vi "Shell.vi"(1 "b":dbl=2.0, 2 "a":dbl=4.0) -> (0 "result":dbl=4.0)   [LabVIEW 2019, in "lv-providershell-example1.lvlib"]
uses:
  lv-providershell-example1.lvlib
  src/VIProviderShellHelper.lvclass
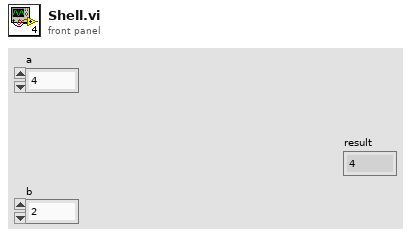
[diagram p1: front panel]
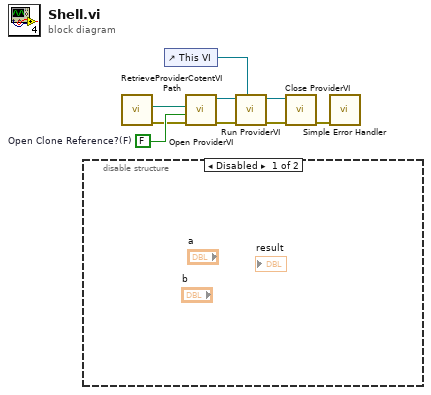
[diagram p0: block diagram]
diagram:
  w5 = FALSE  # Open Clone Reference?(F)
  n1 = disable-structure shown="Disabled" {
    frame Disabled {
    }
    frame Enabled {
    }
  }
  n2 = call "RetrieveProviderCotentVIPath.vi"() -> ("error out"=w1:errorcluster, "Initialize-API"=w2:path)  [unwired: 10 in]
  n3 = control-ref of="This VI"() -> (w4:refnum<vi>)
  n4 = call "Open ProviderVI.vi"("error in (no error)"=w1, "Open Clone Reference?(F)"=w5, "vi path"=w2) -> ("error out"=w7:errorcluster, "vi reference"=w3:refnum<vi>)  [unwired: 7 in]
  n5 = call "Run ProviderVI.vi"("Shell VI"=w4, "error in (no error)"=w7, "vi reference"=w3) -> ("error out"=w8:errorcluster, "VI out"=w9:refnum<vi>)  [unwired: 7 in]
  n6 = call "Close ProviderVI.vi"("error in (no error)"=w8, "VI in"=w9) -> ("error out"=w6:errorcluster)  [unwired: 9 in]
  n7 = call <vilib>:"Simple Error Handler.vi"("error in (no error)"=w6) -> ()  [unwired: 4 in, 5 out]
